vi "Add multiple ROI overlays.vi"(6 "[ROI index] (unity based)":i32[](array[numeric]), 7 "# of Z-planes":i32, 8 "error in":errorcluster, 9 "[ROI info]":T2[](array[typedef]) {"Apparent Frame Size" format="%#_6f"; "Original FOV (um)" format="%#_6f"; "Pixels per miniscan" format="%#_6f"; "Dwell Time per pixel" format="%#_6f"; "Resolution" format="%#_6f"; "ROI group ID" format="%#_6f"; "Laser Power (%)" format="%#_6f"; "Zoom" format="%#_6f"; "Frame Size" format="%#_6f"; "Number of lines" format="%#_6f"; "Composite ID" format="%#_6f"; "Angle (deg)" format="%#_6f"; "ROI Time (ns)" format="%#_6f"; "ROI ID" format="%#_6f"; "Pixels in ROI" format="%#_6f"; "ROI index" format="%#_6f"; "Z stop" format="%#_6f"; "Y stop" format="%#_6f"; "X stop" format="%#_6f"; "Z start" format="%#_6f"; "X start" format="%#_6f"; "Y start" format="%#_6f"}, 10 "Image 2 in":T1, 11 "Image 1 in":T1) -> (0 "error out":errorcluster, 2 "Image 2 out":T1, 3 "Image 1 out":T1)   [LabVIEW 2020]
uses:
  Typedefs/ROI parameters data type.ctl
  <vilib>/vision/Image Controls.llb/IMAQ Image.ctl
  Global variables/gl_Functional Imaging-Global variables.vi
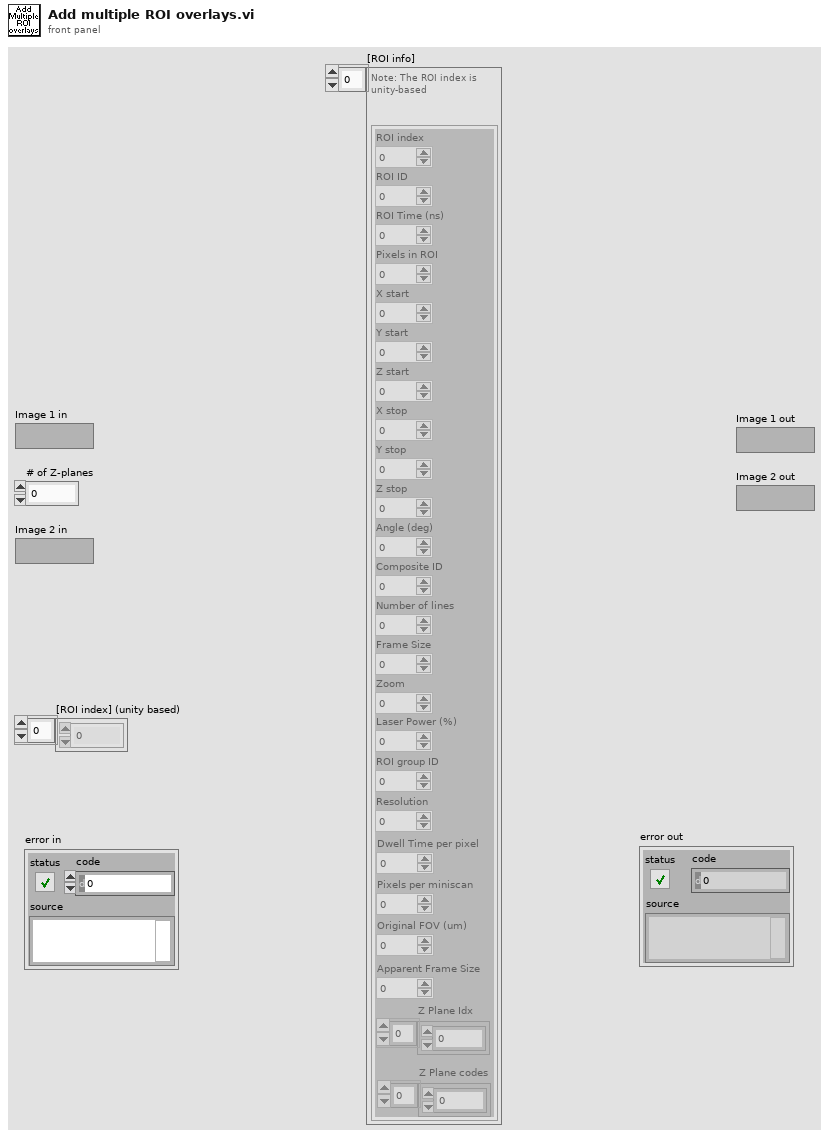
[diagram p1: front panel]
types:
  T1 = typedef "IMAQ Image.ctl" = refnum<image>
  T2 = typedef "ROI parameters data type.ctl" = cluster{"ROI index":dbl, "ROI ID":dbl, "ROI Time (ns)":dbl, "Pixels in ROI":dbl, "X start":dbl, "Y start":dbl, "Z start":dbl, "X stop":dbl, "Y stop":dbl, "Z stop":dbl, "Angle (deg)":dbl, "Composite ID":dbl, "Number of lines":dbl, "Frame Size":dbl, "Zoom":dbl, "Laser Power (%)":dbl, "ROI group ID":dbl, "Resolution":dbl, "Dwell Time per pixel":dbl, "Pixels per miniscan":dbl, "Original FOV (um)":dbl, "Apparent Frame Size":dbl, "Z Plane Idx":i32[], "Z Plane codes":i32[]}
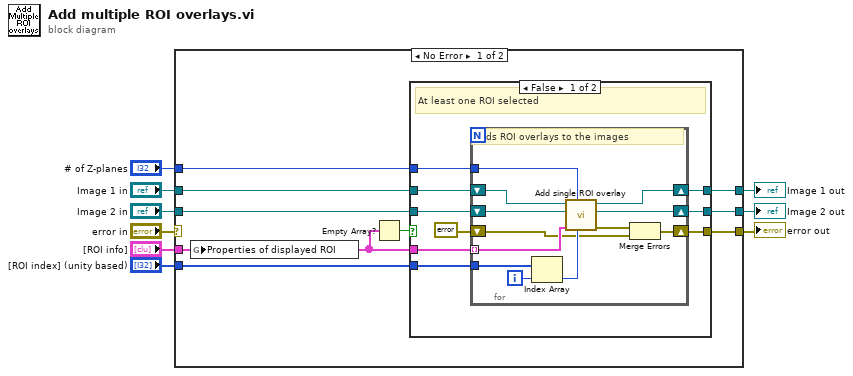
[diagram p0: block diagram]
diagram:
  n1 = case shown="No Error" "error in" {
    selector: "error in" -> [_ w44]
    tunnel: "[ROI index] (unity based)" -> [w18 _]
    tunnel: "# of Z-planes" -> [w17 _]
    tunnel: [w16 w42] -> w7
    tunnel: "Image 2 in" -> [w15 w42]
    tunnel: [w14 w43] -> w5
    tunnel: "Image 1 in" -> [w13 w43]
    tunnel: "[ROI info]" -> [w10 _]
    tunnel: [w11 w44] -> w1
    frame No Error {
      n2 = global write "gl_Functional Imaging-Global variables.vi" "Properties of displayed ROI"(w10) -> ()
      n3 = Empty Array?(array=w10) -> (empty?=w12:bool)
      n4 = case shown="False" w12 {
        tunnel: w18 -> [w27 _]
        tunnel: w10 -> [w26 _]
        tunnel: w17 -> [w25 _]
        tunnel: [w24 w40] -> w16
        tunnel: w15 -> [w23 w40]
        tunnel: [w22 w41] -> w14
        tunnel: w13 -> [w21 w41]
        tunnel: [w19 _] -> w11
        frame False {
          # "At least one ROI selected"
          n5 = for {
            shift-right: [w35] -> w24
            shift-left: w23 -> [w36]
            shift-right: [w39] -> w22
            shift-left: w21 -> [w38]
            tunnel: w26 -> [w37] mode=indexing
            tunnel: w25 -> [w34]
            tunnel: w27 -> [w33]
            shift-right: [w29] -> w19
            shift-left: errorcluster {"status"=FALSE, "code"=0, "source"=""} ("error IO") -> [w28]
            i -> [w32]
            # "Adds ROI overlays to the images"
            n6 = Index Array(array=w33, index=w32) -> (element=w31:i32)
            n7 = call "Add single ROI overlay.vi"("Abs. index of selected Z-plane (unity-based)"=w31, "Number of Z-planes"=w34, "ROI Properties"=w37, "Image2"=w36, "Image1"=w38) -> ("Error out"=w30:errorcluster, "Image2 Out"=w35:T1, "Image1 Out"=w39:T1)  [unwired: 4 in]
            n8 = Merge Errors(w30, w28) -> (w29:errorcluster)
          }
        }
        frame True {
          # "No ROI selected"
        }
      }
    }
    frame Error {
    }
  }
  "Image 2 out" <- w7
  "Image 1 out" <- w5
  "error out" <- w1
